vi "MACH_LightDrive_Colors.vi"(8 "Bank4 Color":u32(colorbox), 9 "Bank3 Color":u32(colorbox), 10 "Bank2 Color":u32(colorbox), 11 "Bank1 Color":u32(colorbox)) -> (2 "Raw Levels":u8[](array[numeric]))   [LabVIEW 2016]
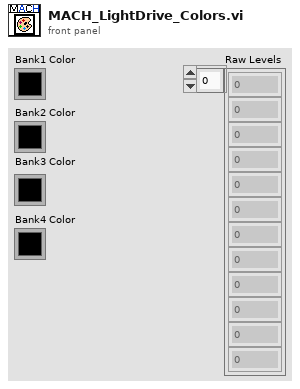
[diagram p1: front panel]
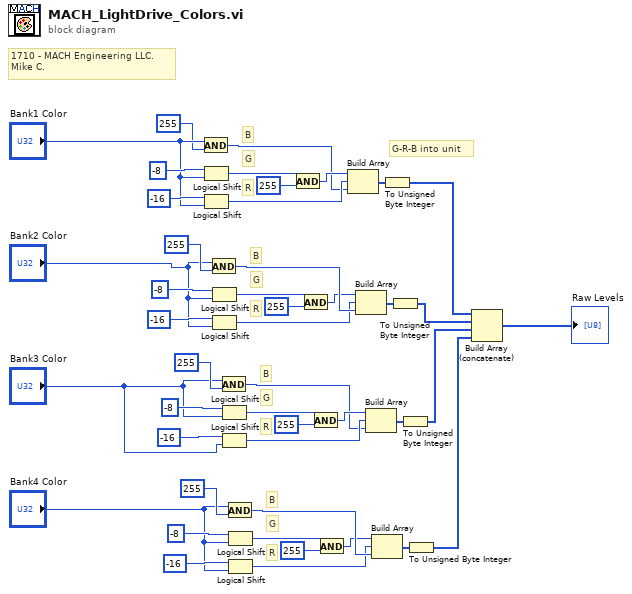
[diagram p0: block diagram]
diagram:
  # "B"
  # "G"
  # "R"
  # "B"
  # "G"
  # "R"
  # "B"
  # "G"
  # "R"
  # "B"
  # "G"
  # "R"
  # "G-R-B into unit"
  # "1710 - MACH Engineering LLC.\nMike C."
  n1 = And(x="Bank1 Color", y=u32 255) -> (x .and. y?=w34:u32)
  n2 = Logical Shift(y=i16 -8, x="Bank1 Color") -> (x << y=w43:u32)
  n3 = Logical Shift(y=i16 -16, x="Bank1 Color") -> (x << y=w35:u32)
  n4 = And(x="Bank2 Color", y=u32 255) -> (x .and. y?=w33:u32)
  n5 = Logical Shift(y=i16 -8, x="Bank2 Color") -> (x << y=w27:u32)
  n6 = Logical Shift(y=i16 -16, x="Bank2 Color") -> (x << y=w32:u32)
  n7 = And(x="Bank3 Color", y=u32 255) -> (x .and. y?=w16:u32)
  n8 = Logical Shift(y=i16 -8, x="Bank3 Color") -> (x << y=w22:u32)
  n9 = Logical Shift(y=i16 -16, x="Bank3 Color") -> (x << y=w17:u32)
  n10 = And(x="Bank4 Color", y=u32 255) -> (x .and. y?=w15:u32)
  n11 = Logical Shift(y=i16 -8, x="Bank4 Color") -> (x << y=w9:u32)
  n12 = Logical Shift(y=i16 -16, x="Bank4 Color") -> (x << y=w14:u32)
  n13 = And(x=w43, y=u32 255) -> (x .and. y?=w36:u32)
  n14 = And(x=w27, y=u32 255) -> (x .and. y?=w31:u32)
  n15 = And(x=w22, y=u32 255) -> (x .and. y?=w18:u32)
  n16 = And(x=w9, y=u32 255) -> (x .and. y?=w13:u32)
  n17 = Build Array(w36, w35, w34) -> (w38:u32[])
  n18 = Build Array(w31, w32, w33) -> (w30:u32[])
  n19 = Build Array(w18, w17, w16) -> (w19:u32[])
  n20 = Build Array(w13, w14, w15) -> (w12:u32[])
  n21 = To Unsigned Byte Integer(number=w38) -> (unsigned 8bit integer=w37:u8[])
  n22 = To Unsigned Byte Integer(number=w30) -> (unsigned 8bit integer=w3:u8[])
  n23 = To Unsigned Byte Integer(number=w19) -> (unsigned 8bit integer=w2:u8[])
  n24 = To Unsigned Byte Integer(number=w12) -> (unsigned 8bit integer=w1:u8[])
  n25 = Build Array (concatenate)(w37, w3, w2, w1) -> (→"Raw Levels":u8[])
